vi "setRunState.vi"(8 "error in (no error)":errorcluster, 10 "Runstate":T1, 11 "ScopeNi in":refnum<class "ScopeNi.lvclass">) -> (0 "error out":errorcluster, 3 "ScopeNi out":refnum<class "ScopeNi.lvclass">)   [LabVIEW 2023, in "ScopeNi.lvclass"]
doc: "<b>Author:</b> Wolfgang\n<b>Description:</b> Set Scope Runstate."
uses:
  ScopeNi.lvclass
  Data/scopeRunState.ctl
  ScopeNi.lvclass/ScopeNi.ctl
  sweScope.lvlib
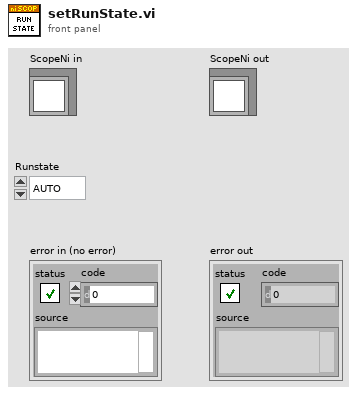
[diagram p1: front panel]
types:
  T1 = typedef "sweScope.lvlib/scopeRunState.ctl" = enum16{"AUTO", "NORMAL", "SINGLE"}
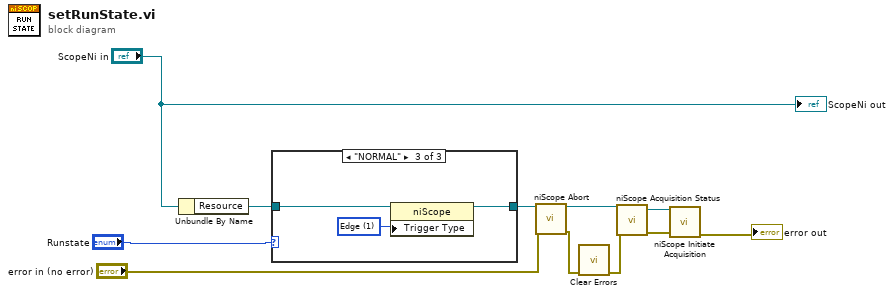
[diagram p0: block diagram]
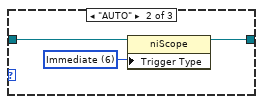
[diagram p3: hidden frame]
diagram:
  n1 = Unbundle By Name("ScopeNi in") -> ("Resource"=w10:refnum<k15>)
  n2 = case shown="\"NORMAL\"" "Runstate" {
    tunnel: w10 -> [w12 w15 w18]
    tunnel: [w12 w14 w17] -> w2
    frame Default {
    }
    frame "AUTO" {
      w13 = 6 items=["Edge"=1, "Width"=2, "Runt"=3, "Glitch"=4, "Video"=5, "Immediate"=6, "Hysteresis"=1001, "Digital"=1002, "Window"=1003, "Software"=1004] ("Triggering:Trigger Type")
      n3 = property class="niScope"(reference=w15, "Trigger Type"=w13) -> (reference out=w14:refnum<k15>)  [unwired: 1 in, 1 out]
    }
    frame "NORMAL" {
      w16 = 1 items=["Edge"=1, "Width"=2, "Runt"=3, "Glitch"=4, "Video"=5, "Immediate"=6, "Hysteresis"=1001, "Digital"=1002, "Window"=1003, "Software"=1004] ("Triggering:Trigger Type")
      n4 = property class="niScope"(reference=w18, "Trigger Type"=w16) -> (reference out=w17:refnum<k15>)  [unwired: 1 in, 1 out]
    }
  }
  n5 = call <instrlib>:"niScope Abort.vi"("instrument handle"=w2, "error in"="error in (no error)") -> ("instrument handle out"=w9:refnum<k15>, "error out"=w8:errorcluster)  [unwired: 12 in]
  n6 = call <vilib>:"Clear Errors.vi"("error in (no error)"=w8) -> ("error out"=w7:errorcluster)  [unwired: 5 in, 1 out]
  n7 = call <instrlib>:"niScope Acquisition Status.vi"("instrument handle"=w9, "error in"=w7) -> ("instrument handle out"=w11:refnum<k15>, "error out"=w6:errorcluster)  [unwired: 11 in, 1 out]
  n8 = call <instrlib>:"niScope Initiate Acquisition.vi"("instrument handle"=w11, "error in"=w6) -> ("error out"=→"error out":errorcluster)  [unwired: 12 in, 1 out]
  "ScopeNi out" <- "ScopeNi in"
